vi "Config Waveform.vi"(0 "VISA resource name":refnum<visa-resource-name>, 1 "End Point (1000)":u32=1000 max=4000000 step=1, 2 "Start Point (0)":u32 max=4000000 step=1, 5 "Select Trace (1)":u16=1 min=1 max=8 step=1, 11 "error in (no error)":errorcluster) -> (4 "VISA resource name out":refnum<visa-resource-name>, 15 "error out":errorcluster)   [LabVIEW 2013, in "Yokogawa PZ4000.lvlib"]
doc: "This VI sends the Waveform Configuration Commands from the PZ4000 series.\nWaveform Configuration Functions are Select Trace, Start Point and End Point"
uses:
  <instrlib>/Yokogawa PZ4000/Yokogawa PZ4000.lvlib
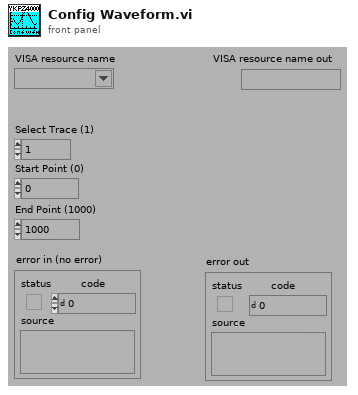
[diagram p1: front panel]
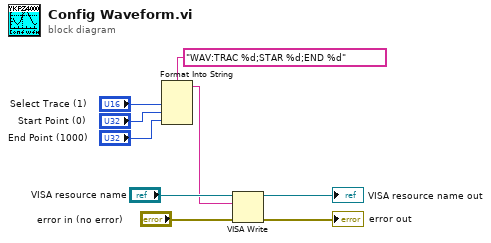
[diagram p0: block diagram]
diagram:
  n1 = Format Into String(format string="WAV:TRAC %d;STAR %d;END %d", "Select Trace (1)", "Start Point (0)", "End Point (1000)") -> (resulting string=w1:string)  [unwired: 2 in, 1 out]
  n2 = VISA Write(VISA resource name="VISA resource name", write buffer=w1, error in (no error)="error in (no error)") -> (VISA resource name out=→"VISA resource name out":refnum<visa-resource-name>, error out=→"error out":errorcluster)  [unwired: 1 out]
